vi "Step Counter.Start Section.vi"(1 "Step State":T1) -> (0 "Step State Out":T1)   [LabVIEW 2018]
uses:
  Step Counter.State Info.ctl
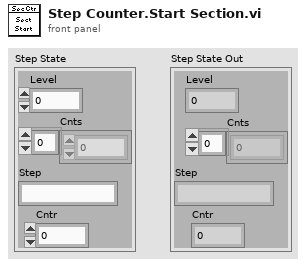
[diagram p1: front panel]
types:
  T1 = typedef "Step Counter.State Info.ctl" = cluster{"Level":i32, "Cnts":i32[], "Step":string, "Cntr":i32}
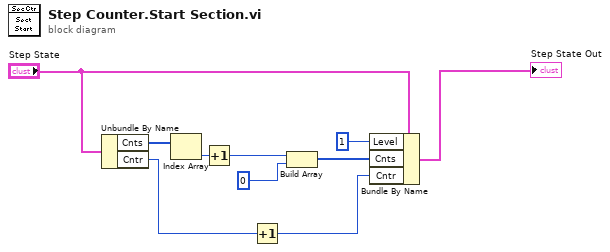
[diagram p0: block diagram]
diagram:
  n1 = Unbundle By Name("Step State") -> ("Cnts"=w10:i32[], "Cntr"=w2:i32)
  n2 = Index Array(array=w10) -> (element=w9:i32)  [unwired: 1 in]
  n3 = Increment(x=w9) -> (x+1=w8:i32)
  n4 = Increment(x=w2) -> (x+1=w1:i32)
  n5 = Build Array(w8, 0 ("element")) -> (w5:i32[])
  n6 = Bundle By Name(cluster="Step State", "Level"=1 ("element"), "Cnts"=w5, "Cntr"=w1) -> (→"Step State Out":T1)
